vi "Set Syringe-Line Valve.vi"(8 "error in (no error)":errorcluster, 9 "Interlock Chain":refnum<class "Interlock Chain.lvclass">, 10 "ON/OFF(OFF)":bool, 11 "cRIO-CO2 in":refnum<class "cRIO-CO2.lvclass">) -> (0 "error out":errorcluster, 3 "cRIO-CO2 out":refnum<class "cRIO-CO2.lvclass">)   [LabVIEW 2015, in "cRIO-Carbondioxide.lvlib" / "cRIO-CO2.lvlib" / "cRIO-CO2.lvclass"]
uses:
  cRIO-CO2.lvclass
  Interlocks/Interlock Chain/Interlock Chain.lvclass
  cRIO-CO2.lvclass/cRIO-CO2.ctl
  Syringe Line Messages/Set Syringe Valve/Set Valve Msg/Set Syringe Valve Msg.lvclass/Set Syringe Valve Msg.ctl
  <vilib>/ActorFramework/Message Enqueuer/Message Enqueuer.lvclass/Message Enqueuer.ctl
  <vilib>/ActorFramework/Message Enqueuer/Enqueue.vi
  <vilib>/ActorFramework/Message Priority Queue/Priority Enqueue.vi
  Syringe Line Messages/Set Syringe Valve/Set Valve Msg/Set Syringe Valve Msg.lvclass
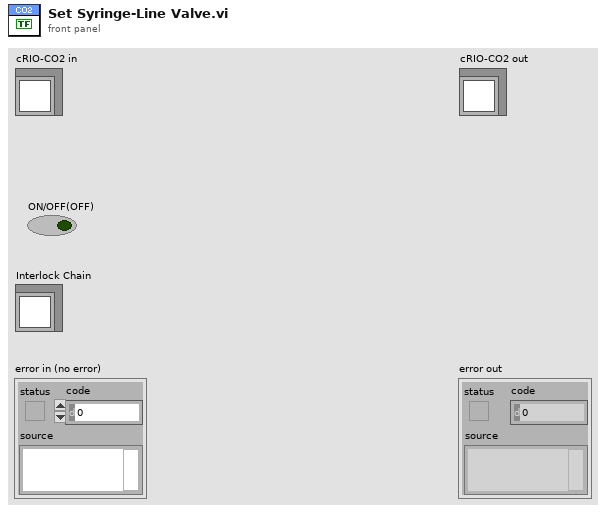
[diagram p1: front panel]
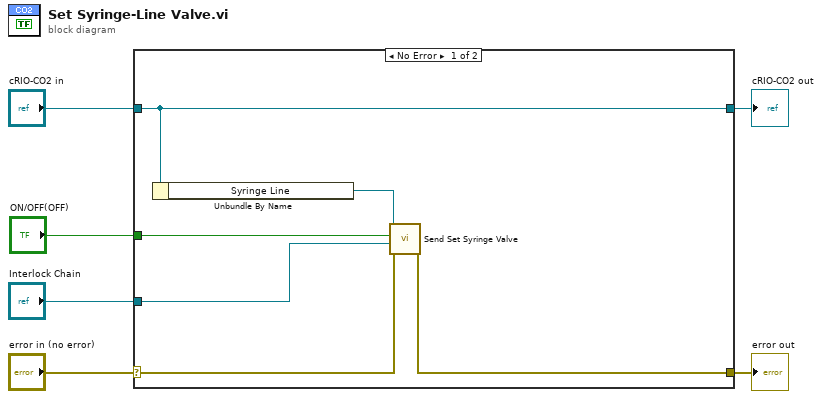
[diagram p0: block diagram]
diagram:
  n1 = case shown="No Error" "error in (no error)" {
    selector: "error in (no error)" -> [w10 w14]
    tunnel: [w9 w14] -> w5
    tunnel: [w12 w13] -> w3
    tunnel: "cRIO-CO2 in" -> [w12 w13]
    tunnel: "ON/OFF(OFF)" -> [w8 _]
    tunnel: "Interlock Chain" -> [w7 _]
    frame No Error {
      n2 = Unbundle By Name(w12) -> ("Syringe Line"=w11:refnum<class "Message Enqueuer.lvclass">)
      n3 = call "Send Set Syringe Valve.vi"("error in (no error)"=w10, "Interlock Chain.lvclass"=w7, "Open? (False)"=w8, "Message Enqueuer"=w11) -> ("error out"=w9:errorcluster)  [unwired: 6 in, 1 out]
    }
    frame Error {
    }
  }
  "error out" <- w5
  "cRIO-CO2 out" <- w3
